vi "VisionDashWrite.vi"(8 "MaxAmbiguity":dbl, 9 "InitialOrientationDeg":dbl, 10 "InitialYPositionFt":dbl, 11 "InitialXPositionFt":dbl) -> ()   [LabVIEW 2023]
doc: "Vision Network\n\nInput\n --Error in \n\nOutput\n --Error out"
uses:
  <vilib>/Rock Robotics/WPI/ThirdParty/JAS_Junk/TrajLib/Rotation2d_CreateAngle.vi
  <vilib>/Rock Robotics/WPI/ThirdParty/JAS_Junk/TrajLib/Translation2d_Create.vi
  <vilib>/Rock Robotics/Network Tables/NT Write Number.vi
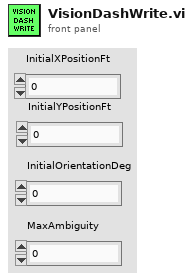
[diagram p1: front panel]
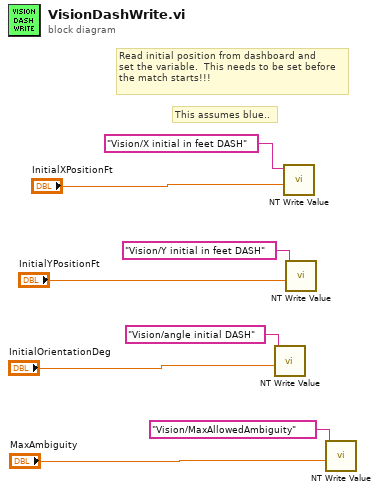
[diagram p0: block diagram]
diagram:
  # "This assumes blue.."
  # "Read initial position from dashboard and\nset the variable.  This needs to be set before\nthe match starts!!!"
  n1 = call-poly <vilib>:"NT Write Value.vi"("value"="InitialOrientationDeg", "name"="Vision/angle initial DASH") -> ()  [unwired: 9 in, 1 out]
  n2 = call-poly <vilib>:"NT Write Value.vi"("value"="InitialXPositionFt", "name"="Vision/X initial in feet DASH") -> ()  [unwired: 9 in, 1 out]
  n3 = call-poly <vilib>:"NT Write Value.vi"("value"="InitialYPositionFt", "name"="Vision/Y initial in feet DASH") -> ()  [unwired: 9 in, 1 out]
  n4 = call-poly <vilib>:"NT Write Value.vi"("value"="MaxAmbiguity", "name"="Vision/MaxAllowedAmbiguity") -> ()  [unwired: 9 in, 1 out]
